vi "getConnectionPoint.vi"(0 "reference":refnum<class "CallNode.lvclass">, 1 "direction":refnum<class "Direction.lvclass">, 5 "error in (no error)":errorcluster) -> (14 "reference out":refnum<class "CallNode.lvclass">, 15 "point2D":T1 {"y" format="%.2f"; "x" format="%.2f"}, 19 "error out":errorcluster)   [LabVIEW 2012, in "CallNode.lvclass"]
doc: "public Point2D getConnectionPoint(Direction d)"
uses:
  <resource>/Framework/Providers/Open_GDS/UML/CallNode_class/CallNode.lvclass
  <resource>/Framework/Providers/Open_GDS/UML/Direction_class/Direction.lvclass
  <resource>/Framework/Providers/Open_GDS/UML/General/Point/Point Point2D.ctl
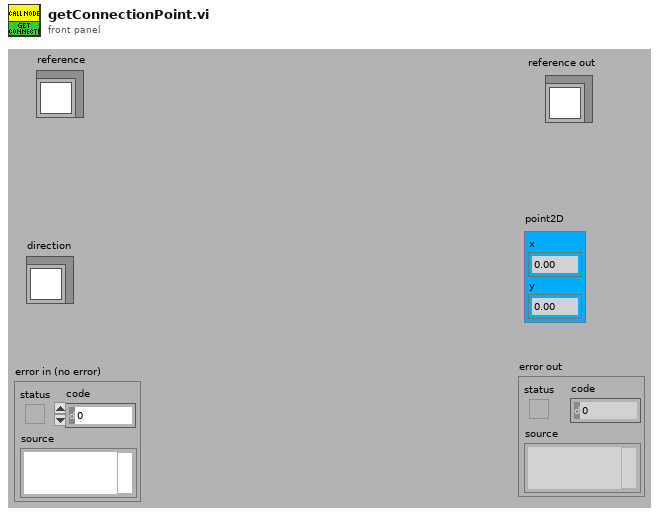
[diagram p1: front panel]
types:
  T1 = typedef "Point Point2D.ctl" = cluster{"x":dbl, "y":dbl}
  T2 = typedef "CallNode.lvclass/ObjectAttributes.ctl" = cluster{"Base class":T3, "objectCallNodeRef":refnum<class "AbstractNode.lvclass">, "signaled":bool, "openBottom":bool, "DEFAULT_WIDTH":i32, "DEFAULT_HEIGHT":i32, "CALL_YGAP":i32}
  T3 = typedef "RectangularNode.lvclass/ObjectAttributes.ctl" = cluster{"Base class":T4, "bounds":T5}
  T4 = typedef "AbstractNode.lvclass/ObjectAttributes.ctl" = cluster{"parent":refnum<class "AbstractNode.lvclass">, "children":refnum<class "AbstractNode.lvclass">[], "Hidden":bool}
  T5 = typedef "Rectangle Rectangle2D.ctl" = cluster{"x":dbl, "y":dbl, "width":dbl, "height":dbl}
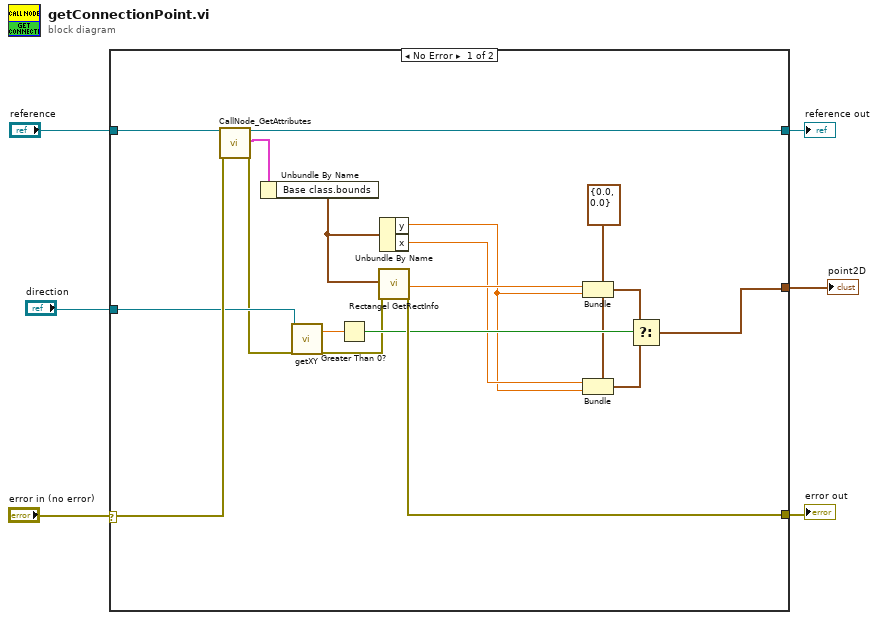
[diagram p0: block diagram]
diagram:
  n1 = case shown="No Error" "error in (no error)" {
    selector: "error in (no error)" -> [w21 w25]
    tunnel: "reference" -> [w24 w26]
    tunnel: [w23 w25] -> w5
    tunnel: [w22 w26] -> w4
    tunnel: "direction" -> [w20 _]
    tunnel: [w19 _] -> w1
    frame No Error {
      w16 = T1 {"x"=0.0, "y"=0.0} ("point2D")
      n2 = call <resource>:"CallNode_GetAttributes.vi"("reference in"=w24, "error in (no error)"=w21) -> ("reference out"=w22:refnum<class "CallNode.lvclass">, "Attributes"=w10:T2, "error out"=w8:errorcluster)  [unwired: 15 out]
      n3 = Unbundle By Name(w10) -> ("Base class.bounds"=w13:T5)
      n4 = call <resource>:"getXY.vi"("reference"=w20, "error in (no error)"=w8) -> ("x"=w18:dbl, "error out"=w9:errorcluster)  [unwired: 16 out]
      n5 = Greater Than 0?(x=w18) -> (x > 0?=w17:bool)
      n6 = call <resource>:"Rectangel GetRectInfo.vi"("bounds"=w13, "error in (no error)"=w9) -> ("maxX"=w14:dbl, "error out"=w23:errorcluster)  [unwired: 16 out]
      n7 = Unbundle By Name(w13) -> ("y"=w7:dbl, "x"=w11:dbl)
      n8 = Bundle(cluster=w16, "x"=w14, "y"=w7) -> (w15:T1)
      n9 = Bundle(cluster=w16, "x"=w11, "y"=w7) -> (w12:T1)
      n10 = Select(t=w15, s=w17, f=w12) -> (s? t:f=w19:T1)
    }
    frame Error {
    }
  }
  "reference out" <- w4
  "error out" <- w5
  "point2D" <- w1
